vi "Load Child Method.vi"() -> ()   [LabVIEW 2020, in "MacroAssert.lvlib"]
uses:
  MacroAssert.lvlib
  Classes/Step/Step.lvclass
  CTLs/Step Type V3.ctl
panel:
  in  "Step Type":T1
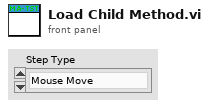
[diagram p1: front panel]
types:
  T1 = typedef "MacroAssert.lvlib/Step Type V3.ctl" = enum16{"Mouse Move", "Mouse Click", "Key Press", "Wait", "Mouse Down", "Mouse Up", "Key Down", "Key Up", "Maximize Window", "Restore Window", "Minimize Window", "Close Window", "Bring Window to Front", "Send Window to Back", "Assertion: Ctl Visible", "Assertion: Ctl Disabled", "Assertion: Ctl Image"}
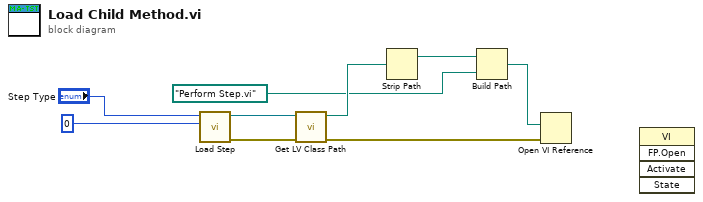
[diagram p0: block diagram]
diagram:
  n1 = call "Load Step.vi"("Index"=0, "Step Type"="Step Type") -> ("error out"=w2:errorcluster, "Step"=w7:refnum<class "Step.lvclass">)  [unwired: 8 in]
  n2 = call <vilib>:"Get LV Class Path.vi"("error in (no error)"=w2, "object"=w7) -> ("error out"=w1:errorcluster, "class path"=w6:path)  [unwired: 8 in]
  n3 = Strip Path(path=w6) -> (stripped path=w5:path)  [unwired: 1 out]
  n4 = Build Path(base path=w5, name or relative path=path "Perform Step.vi") -> (appended path=w3:path)
  n5 = Open VI Reference(vi path=w3, error in (no error)=w1) -> ()  [unwired: 4 in, 2 out]
  n6 = invoke class="VI" method="FP.Open"() -> ()  [unwired: 5 in, 5 out]
